vi "Init.vi"(8 "error in (no error)":errorcluster, 11 "Mock In":refnum<class "Pure Mock.lvclass">) -> (0 "error out":errorcluster, 3 "Mock Out":refnum<class "Pure Mock.lvclass">)   [LabVIEW 2020, in "Pure Mock.lvclass"]
uses:
  Pure Mock.lvclass
  Core/Expectation/Expectation.lvclass
  Pure Mock.lvclass/Pure Mock.ctl
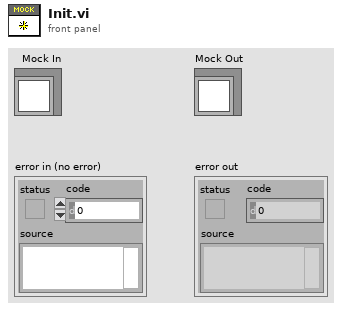
[diagram p1: front panel]
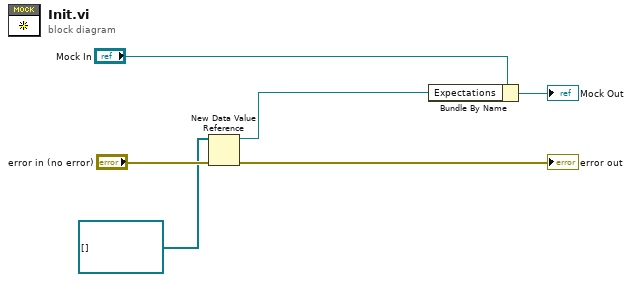
[diagram p0: block diagram]
diagram:
  n1 = New Data Value Reference(data value=refnum<class "Expectation.lvclass">[] [] ("Array"), error in="error in (no error)") -> (data value reference=w2:refnum<data-value>, error out=→"error out":errorcluster)
  n2 = Bundle By Name(cluster="Mock In", "Expectations"=w2) -> (→"Mock Out":refnum<class "Pure Mock.lvclass">)
